vi "Tosca-Start DI Thread.vi"(0 "DI":refnum<queue>, 5 "Input Events":T4[](array[typedef]), 7 "Imaging":T2, 9 "Action":enum16{"Stop", "Preview", "Run"}(ring)=enum."Preview", 11 "error in (no error)":errorcluster, 12 "Flags":T1[](array[typedef])) -> (15 "error out":errorcluster)   [LabVIEW 2020]
uses:
  Tosca-Input Event.ctl
  Tosca-Input Criterion.ctl
  epl-vi-lib/Utility VIs/Type Defs/Logic State.ctl
  Typedefs/Tosca-Accumulator.ctl
  Typedefs/Tosca-Imaging.ctl
  Imaging VIs/Tosca-Imaging Mode.ctl
  Tosca-DI Queue Data.ctl
  Typedefs/Tosca-Flag.ctl
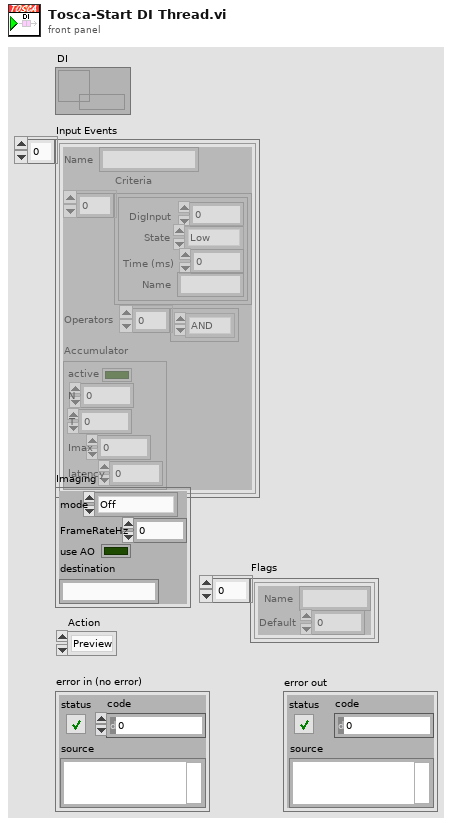
[diagram p1: front panel]
types:
  T1 = typedef "Tosca-Flag.ctl" = cluster{"Name":string, "Default":i32}
  T2 = typedef "Tosca-Imaging.ctl" = cluster{"mode":T3, "FrameRateHz":dbl, "use AO":bool, "destination":string}
  T3 = typedef "Tosca-Imaging Mode.ctl" = enum16{"Off", "Widefield", "Two-photon"}
  T4 = typedef "Tosca-Input Event.ctl" = cluster{"Name":string, "Criteria":T5[], "Operators":enum16{"AND", "OR"}[], "Accumulator":T7}
  T5 = typedef "Tosca-Input Criterion.ctl" = cluster{"DigInput":i32, "State":T6, "Time (ms)":i32, "Name":string}
  T6 = typedef "Logic State.ctl" = enum16{"Low", "High", "Rising", "Falling"}
  T7 = typedef "Tosca-Accumulator.ctl" = cluster{"active":bool, "N":i32, "T":dbl, "Imax":dbl, "latency":dbl}
  T8 = typedef "Tosca-DI Queue Data.ctl" = cluster{"Action":enum16{"Stop", "Preview", "Run"}, "Input Events":T4[]}
  T9 = cluster{"Action":enum16{"Stop", "Preview", "Run"}, "Input Events Out":T4[]}
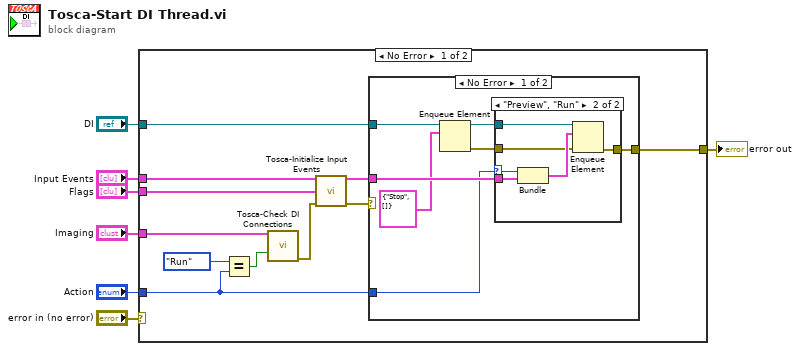
[diagram p0: block diagram]
diagram:
  n1 = case shown="No Error" "error in (no error)" {
    selector: "error in (no error)" -> [_ w34]
    tunnel: "Input Events" -> [w15 _]
    tunnel: "Imaging" -> [w14 _]
    tunnel: [w13 w34] -> w4
    tunnel: "DI" -> [w12 _]
    tunnel: "Action" -> [w9 _]
    tunnel: "Flags" -> [w8 _]
    frame No Error {
      n2 = Equal?(x=enum16{"Stop", "Preview", "Run"}."Run", y=w9) -> (x = y?=w10:bool)
      n3 = call "Tosca-Check DI Connections.vi"("Imaging"=w14, "Include required"=w10) -> ("error out"=w16:errorcluster)  [unwired: 13 in]
      n4 = call "Tosca-Initialize Input Events.vi"("Input Events"=w15, "Flags"=w8, "error in (no error)"=w16) -> ("Input Events Out"=w18:T4[], "error IO"=w17:errorcluster)  [unwired: 11 in]
      n5 = case shown="No Error" w17 {
        selector: w17 -> [_ w33]
        tunnel: w12 -> [w20 _]
        tunnel: w18 -> [w25 _]
        tunnel: [w21 w33] -> w13
        tunnel: w9 -> [w19 _]
        frame No Error {
          n6 = Enqueue Element(queue=w20, element=T8 {"Action"=enum."Stop", "Input Events"=[]}) -> (queue out=w24:refnum<queue>, error out=w22:errorcluster)  [unwired: 2 in, 1 out]
          n7 = case shown="\"Preview\", \"Run\"" w19 {
            selector: w19 -> [_ w27]
            tunnel: w25 -> [_ w31]
            tunnel: w24 -> [_ w30]
            tunnel: w22 -> [w26 w29]
            tunnel: [w26 w28] -> w21
            frame "Stop", Default {
            }
            frame "Preview", "Run" {
              n8 = Bundle("Action"=w27, "Input Events Out"=w31) -> (w32:T9)  [unwired: 1 in]
              n9 = Enqueue Element(queue=w30, element=w32, error in (no error)=w29) -> (error out=w28:errorcluster)  [unwired: 1 in, 2 out]
            }
          }
        }
        frame Error {
        }
      }
    }
    frame Error {
    }
  }
  "error out" <- w4
